vi "Control_2.vi"(0 "latd-lon-heig-VNWU":T4, 1 "CIVITA as DMARS [rad]":cluster{"phi":dbl, "theta":dbl, "psi":dbl}, 5 "Wi1-Wbi1-qi1-Euli1":T5, 7 "Civita?":bool, 9 "Mab":T3, 11 "File":dbl[][](array[numeric]), 12 "dt-sim_run-t-i":T2, 14 "Rotation":T1, 15 "sim_running":bool) -> (3 "Pitch Yaw ref [deg]":dbl[](array[numeric]), 4 "TVA_cmd(i+1,:) [deg]":dbl[](array[numeric]), 10 "AoA-Speed-Rocket":cluster{dbl[], dbl[], dbl[]})   [LabVIEW 2017]
uses:
  <vilib>/Analysis/coordinate.llb/Euler Rotation Order.ctl
  <vilib>/Analysis/_algsub.llb/Vector Norm Type.ctl
  <vilib>/Analysis/baseanly.llb/Real A x B.vi
  <vilib>/Analysis/_algsub.llb/Real Vector Norm.vi
  <vilib>/Analysis/Matrix/Numeric/Conversions/Array To Matrix - RA2.vi
  <vilib>/Analysis/Matrix/Numeric/Conversions/Matrix To Array - RM.vi
  <vilib>/Analysis/NI_AALPro.lvlib
  <vilib>/Analysis/Matrix/NI_Matrix.lvlib
  <vilib>/Analysis/NI_AALBase.lvlib
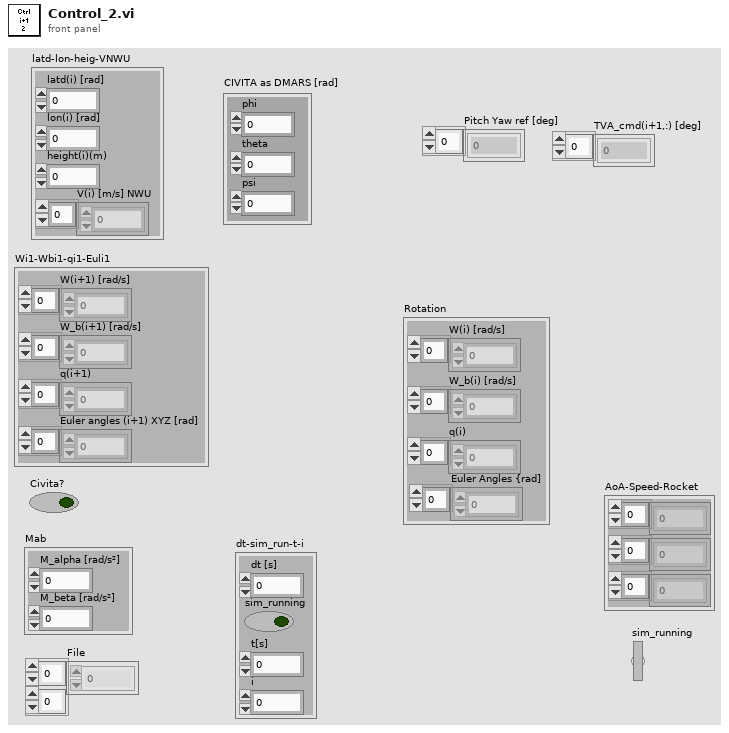
[diagram p1: front panel]
types:
  T1 = cluster{"W(i) [rad/s]":dbl[], "W_b(i) [rad/s]":dbl[], "q(i)":dbl[], "Euler Angles {rad]":dbl[]}
  T2 = cluster{"dt [s]":dbl, "sim_running":bool, "t[s]":dbl, "i":i32}
  T3 = cluster{"M_alpha [rad/s²]":dbl, "M_beta [rad/s²]":dbl}
  T4 = cluster{"latd(i) [rad]":dbl, "lon(i) [rad]":dbl, "height(i)(m)":dbl, "V(i) [m/s] NWU":dbl[]}
  T5 = cluster{"W(i+1) [rad/s]":dbl[], "W_b(i+1) [rad/s]":dbl[], "q(i+1)":dbl[], "Euler angles (i+1) XYZ [rad]":dbl[]}
  T6 = typedef "NI_AALPro.lvlib/Vector Norm Type.ctl" = u16
  T7 = typedef "NI_AALPro.lvlib/Euler Rotation Order.ctl" = u16
  T8 = typedef "NI_Matrix.lvlib/RealMatrix.ctl" = dbl[][]
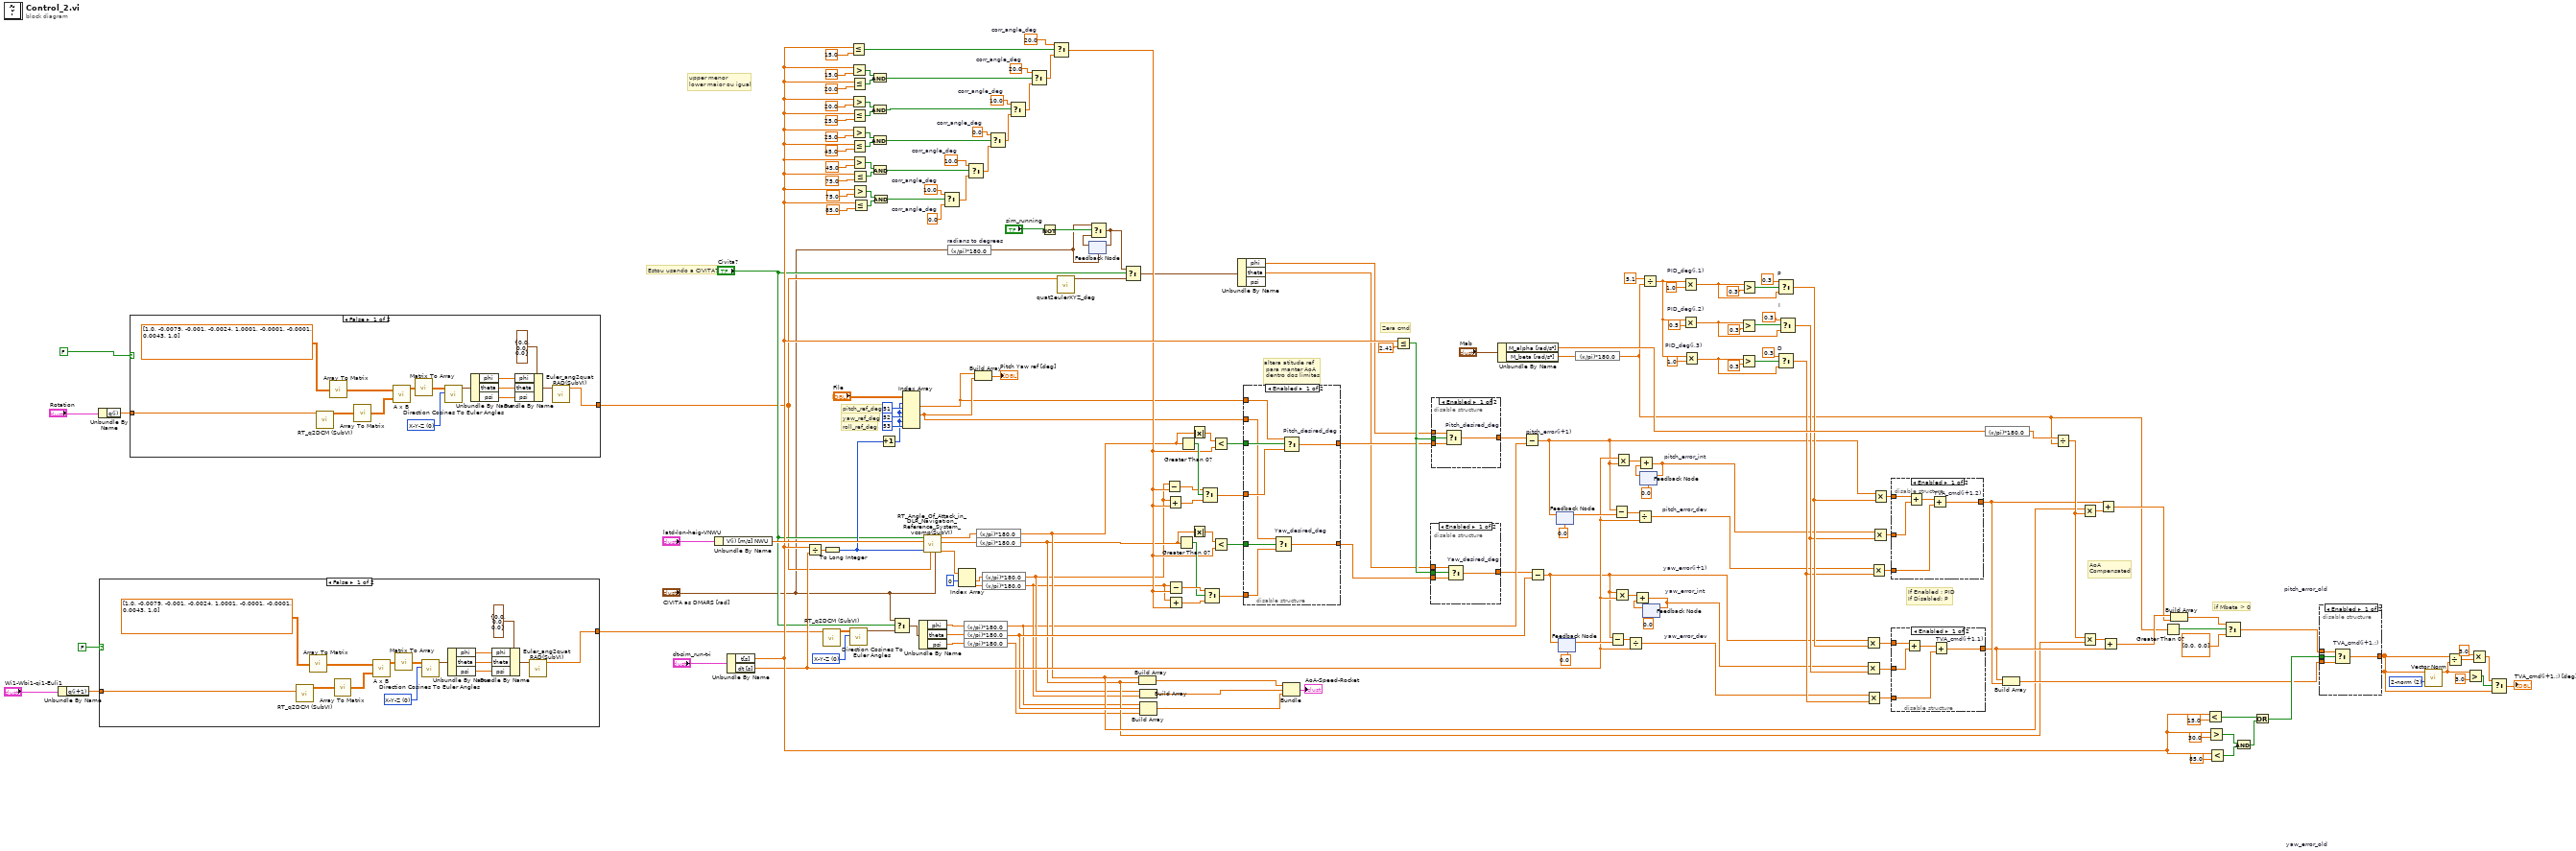
[diagram p0: block diagram]
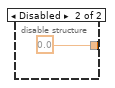
[diagram p5: hidden frame]
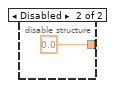
[diagram p8: hidden frame]
diagram:
  w116 = T6 2 items=["1-norm"=1, "2-norm"=2, "Inf-norm"=3, "-Inf-norm"=4, "User Defined"=5] ("norm type")
  w147 = T7 0 items=["X-Y-Z", "X-Z-Y", "Y-X-Z", "Y-Z-X", "Z-X-Y", "Z-Y-X", "X-Y-X", "X-Z-X", "Y-X-Y", "Y-Z-Y", "Z-X-Z", "Z-Y-Z"] ("rotation order")
  w156 = 0.0  # corr_angle_deg
  w159 = 10.0  # corr_angle_deg
  w162 = 10.0  # corr_angle_deg
  w187 = 0.0  # corr_angle_deg
  w189 = 10.0  # corr_angle_deg
  w191 = 20.0  # corr_angle_deg
  w192 = 20.0  # corr_angle_deg
  # "AoA\nCompensated"
  # "Estou usando a CIVITA?"
  # "If Enabled : PID\nIf Disabled: P"
  # "if Mbeta > 0"
  # "altera atitude ref\n para manter AoA\n dentro dos limites"
  # "Zera cmd"
  # "roll_ref_deg"
  # "yaw_ref_deg"
  # "pitch_ref_deg"
  # "upper menor\nlower maior ou igual"
  n1 = Unbundle By Name("Wi1-Wbi1-qi1-Euli1") -> ("q(i+1)"=w8:dbl[])
  n2 = Unbundle By Name("Rotation") -> ("q(i)"=w13:dbl[])
  n3 = case shown="False" FALSE {
    tunnel: w8 -> [w197 w210]
    tunnel: [w196 w210] -> w7
    frame False {
      w208 = T7 0 items=["X-Y-Z", "X-Z-Y", "Y-X-Z", "Y-Z-X", "Z-X-Y", "Z-Y-X", "X-Y-X", "X-Z-X", "Y-X-Y", "Y-Z-Y", "Z-X-Z", "Z-Y-Z"] ("rotation order")
      n4 = call "RT_q2DCM (SubVI).vi"("Quaternion"=w197) -> ("DCM"=w209:dbl[][])  [unwired: 10 in]
      n5 = call-poly <vilib>:"Array To Matrix.vi"("Real 2D Array"=dbl[][] [[1.0, -0.0079, -0.001], [-0.0024, 1.0001, -0.0001], [-0.0001, 0.0043, 1.0]]) -> ("Real Matrix"=w200:T8)
      n6 = call-poly <vilib>:"Array To Matrix.vi"("Real 2D Array"=w209) -> ("Real Matrix"=w199:T8)
      n7 = call-poly <vilib>:"A x B.vi"("B"=w199, "A"=w200) -> ("A x B"=w201:T8)  [unwired: 1 out]
      n8 = call-poly <vilib>:"Matrix To Array.vi"("Real Matrix"=w201) -> ("Real 2D Array"=w202:dbl[][])
      n9 = call <vilib>:"Direction Cosines To Euler Angles.vi"("rotation order"=w208, "Direction Cosines"=w202) -> ("Euler Angles"=w203:cluster{"phi":dbl, "theta":dbl, "psi":dbl})  [unwired: 8 in, 1 out]
      n10 = Unbundle By Name(w203) -> ("phi"=w206:dbl, "theta"=w207:dbl, "psi"=w195:dbl)
      n11 = Bundle By Name(cluster=cluster{"phi":dbl, "theta":dbl, "psi":dbl} {"phi"=0.0, "theta"=0.0, "psi"=0.0} ("Euler Angles 2"), "phi"=w206, "theta"=w207, "psi"=w195) -> (w204:cluster{"phi":dbl, "theta":dbl, "psi":dbl})
      n12 = call "Euler_ang2quat RAD(SubVI).vi"("Euler Angles [rad]"=w204) -> ("Quaternions"=w196:dbl[])  [unwired: 10 in]
    }
    frame True {
    }
  }
  n13 = case shown="False" FALSE {
    tunnel: w13 -> [w213 w226]
    tunnel: [w212 w226] -> w11
    frame False {
      w224 = T7 0 items=["X-Y-Z", "X-Z-Y", "Y-X-Z", "Y-Z-X", "Z-X-Y", "Z-Y-X", "X-Y-X", "X-Z-X", "Y-X-Y", "Y-Z-Y", "Z-X-Z", "Z-Y-Z"] ("rotation order")
      n14 = call "RT_q2DCM (SubVI).vi"("Quaternion"=w213) -> ("DCM"=w225:dbl[][])  [unwired: 10 in]
      n15 = call-poly <vilib>:"Array To Matrix.vi"("Real 2D Array"=dbl[][] [[1.0, -0.0079, -0.001], [-0.0024, 1.0001, -0.0001], [-0.0001, 0.0043, 1.0]]) -> ("Real Matrix"=w216:T8)
      n16 = call-poly <vilib>:"Array To Matrix.vi"("Real 2D Array"=w225) -> ("Real Matrix"=w215:T8)
      n17 = call-poly <vilib>:"A x B.vi"("B"=w215, "A"=w216) -> ("A x B"=w217:T8)  [unwired: 1 out]
      n18 = call-poly <vilib>:"Matrix To Array.vi"("Real Matrix"=w217) -> ("Real 2D Array"=w218:dbl[][])
      n19 = call <vilib>:"Direction Cosines To Euler Angles.vi"("rotation order"=w224, "Direction Cosines"=w218) -> ("Euler Angles"=w219:cluster{"phi":dbl, "theta":dbl, "psi":dbl})  [unwired: 8 in, 1 out]
      n20 = Unbundle By Name(w219) -> ("phi"=w222:dbl, "theta"=w223:dbl, "psi"=w211:dbl)
      n21 = Bundle By Name(cluster=cluster{"phi":dbl, "theta":dbl, "psi":dbl} {"phi"=0.0, "theta"=0.0, "psi"=0.0} ("Euler Angles 2"), "phi"=w222, "theta"=w223, "psi"=w211) -> (w220:cluster{"phi":dbl, "theta":dbl, "psi":dbl})
      n22 = call "Euler_ang2quat RAD(SubVI).vi"("Euler Angles [rad]"=w220) -> ("Quaternions"=w212:dbl[])  [unwired: 10 in]
    }
    frame True {
    }
  }
  n23 = Unbundle By Name("latd-lon-heig-VNWU") -> ("V(i) [m/s] NWU"=w83:dbl[])
  n24 = Unbundle By Name("dt-sim_run-t-i") -> ("t[s]"=w77:dbl, "dt [s]"=w58:dbl)
  n25 = Divide(x=w77, y=w58) -> (x/y=w154:dbl)
  n26 = call "RT_q2DCM (SubVI).vi"("Quaternion"=w7) -> ("DCM"=w148:dbl[][])  [unwired: 10 in]
  n27 = To Long Integer(number=w154) -> (32bit integer=w72:i32)
  n28 = Less Or Equal?(x=w77, y=15.0) -> (x <= y?=w193:bool)
  n29 = call <vilib>:"Direction Cosines To Euler Angles.vi"("rotation order"=w147, "Direction Cosines"=w148) -> ("Euler Angles"=w6:cluster{"phi":dbl, "theta":dbl, "psi":dbl})  [unwired: 8 in, 1 out]
  n30 = Greater?(x=w77, y=15.0) -> (0:w183:bool)
  n31 = Greater?(x=w77, y=20.0) -> (0:w179:bool)
  n32 = Greater?(x=w77, y=25.0) -> (0:w174:bool)
  n33 = Less Or Equal?(x=w77, y=20.0) -> (x <= y?=w182:bool)
  n34 = Less Or Equal?(x=w77, y=25.0) -> (x <= y?=w180:bool)
  n35 = Less Or Equal?(x=w77, y=45.0) -> (x <= y?=w173:bool)
  n36 = Greater?(x=w77, y=45.0) -> (0:w171:bool)
  n37 = Less Or Equal?(x=w77, y=75.0) -> (x <= y?=w172:bool)
  n38 = Greater?(x=w77, y=75.0) -> (0:w166:bool)
  n39 = Less Or Equal?(x=w77, y=85.0) -> (x <= y?=w165:bool)
  n40 = And(x=w183, y=w182) -> (x .and. y?=w181:bool)
  n41 = And(x=w179, y=w180) -> (x .and. y?=w164:bool)
  n42 = And(x=w174, y=w173) -> (x .and. y?=w163:bool)
  n43 = And(x=w171, y=w172) -> (x .and. y?=w161:bool)
  n44 = And(x=w166, y=w165) -> (x .and. y?=w158:bool)
  n45 = Increment(x=w72) -> (x+1=w144:i32)
  n46 = Select(t="CIVITA as DMARS [rad]", s="Civita?", f=w6) -> (s? t:f=w31:cluster{"phi":dbl, "theta":dbl, "psi":dbl})
  n47 = Index Array(array="File", index (row) #1=w144, index (col) #1=51 ("disabled index (col)"), index (row) #2=w144, index (col) #2=52 ("disabled index (col)"), index (row) #3=w144, index (col) #3=53 ("disabled index (col)")) -> (element #1=w36:dbl, element #2=w37:dbl)  [unwired: 1 out]
  n48 = Unbundle By Name(w31) -> ("phi"=w146:dbl, "theta"=w145:dbl, "psi"=w35:dbl)
  n49 = call "RT_Angle_Of_Attack_in_DLR_Navigation_Reference_System_vcomp(SubVI).vi"("Euler Angles [rad]"="CIVITA as DMARS [rad]", "q"=w11, "i"=w72, "V (m/s)"=w83, "Civita?"="Civita?") -> ("Speed_direction [rad]"=w149:dbl[], "AoA_yaw (rad)"=w42:dbl, "AoA_pitch (rad)"=w43:dbl)  [unwired: 4 in]
  n50 = Select(t=w159, s=w158, f=w156) -> (s? t:f=w157:dbl)
  n51 = expression code="(x/pi)*180.0" "radians to degrees"("CIVITA as DMARS [rad]") -> (w17:cluster{"phi":dbl, "theta":dbl, "psi":dbl})
  n52 = Index Array(array=w149, index #1=0 ("index")) -> (element #1=w45:dbl, element #2=w44:dbl)  [unwired: 1 in]
  n53 = expression code="(x/pi)*180.0" ("radians to degrees")(w146) -> (w26:dbl)
  n54 = expression code="(x/pi)*180.0" ("radians to degrees")(w145) -> (w46:dbl)
  n55 = expression code="(x/pi)*180.0" ("radians to degrees")(w35) -> (w34:dbl)
  n56 = Select(t=w162, s=w161, f=w157) -> (s? t:f=w160:dbl)
  n57 = Build Array(w36, w37) -> (→"Pitch Yaw ref [deg]":dbl[])
  n58 = expression code="(x/pi)*180.0" ("radians to degrees")(w43) -> (w41:dbl)
  n59 = expression code="(x/pi)*180.0" ("radians to degrees")(w42) -> (w40:dbl)
  n60 = expression code="(x/pi)*180.0" ("radians to degrees")(w45) -> (w39:dbl)
  n61 = expression code="(x/pi)*180.0" ("radians to degrees")(w44) -> (w38:dbl)
  n62 = Select(t=w187, s=w163, f=w160) -> (s? t:f=w186:dbl)
  n63 = Select(t=w189, s=w164, f=w186) -> (s? t:f=w188:dbl)
  n64 = Select(t=w191, s=w181, f=w188) -> (s? t:f=w190:dbl)
  n65 = Not(x="sim_running") -> (.not. x?=w21:bool)
  n66 = Select(t=w192, s=w193, f=w190) -> (s? t:f=w71:dbl)
  n67 = call "quat2eulerXYZ_deg.vi"("Quaternions"=w11) -> ("Euler Angles [deg]"=w30:cluster{"phi":dbl, "theta":dbl, "psi":dbl})  [unwired: 10 in]
  n68 = feedback #1(w17) -> (w27:cluster{"phi":dbl, "theta":dbl, "psi":dbl})
  n69 = Select(t=w17, s=w21, f=w27) -> (s? t:f=w32:cluster{"phi":dbl, "theta":dbl, "psi":dbl})
  n70 = feedback-in #1(w32) -> ()
  n71 = Select(t=w32, s="Civita?", f=w30) -> (s? t:f=w29:cluster{"phi":dbl, "theta":dbl, "psi":dbl})
  n72 = Build Array(w41, w40) -> (w16:dbl[])
  n73 = Build Array(w39, w38) -> (w15:dbl[])
  n74 = Build Array(w26, w46, w34) -> (w14:dbl[])
  n75 = Subtract(x=w39, y=w71) -> (x-y=w104:dbl)
  n76 = Add(x=w39, y=w71) -> (x+y=w103:dbl)
  n77 = Subtract(x=w38, y=w71) -> (x-y=w101:dbl)
  n78 = Add(x=w38, y=w71) -> (x+y=w102:dbl)
  n79 = Greater Than 0?(x=w40) -> (x > 0?=w100:bool)
  n80 = Greater Than 0?(x=w41) -> (x > 0?=w105:bool)
  n81 = Absolute Value(x=w41) -> (abs(x)=w108:dbl)
  n82 = Absolute Value(x=w40) -> (abs(x)=w97:dbl)
  n83 = Select(t=w104, s=w105, f=w103) -> (s? t:f=w106:dbl)
  n84 = Select(t=w101, s=w100, f=w102) -> (s? t:f=w99:dbl)
  n85 = Less?(x=w108, y=w71) -> (x < y?=w107:bool)
  n86 = Less?(x=w97, y=w71) -> (x < y?=w98:bool)
  n87 = Unbundle By Name(w29) -> ("phi"=w19:dbl, "theta"=w18:dbl)  [unwired: 1 out]
  n88 = disable-structure shown="Enabled" {
    disable-tunnel: w37 -> [w228 w235]
    disable-tunnel: w36 -> [w230 w236]
    disable-tunnel: w107 -> [w234 _]
    disable-tunnel: w106 -> [w229 _]
    disable-tunnel: w99 -> [w227 _]
    disable-tunnel: w98 -> [w231 _]
    disable-tunnel: [w233 w236] -> w94
    disable-tunnel: [w232 w235] -> w93
    frame Enabled {
      n89 = Select "Yaw_desired_deg"(t=w228, s=w231, f=w227) -> (s? t:f=w232:dbl)
      n90 = Select "Pitch_desired_deg"(t=w230, s=w234, f=w229) -> (s? t:f=w233:dbl)
    }
    frame Disabled {
    }
  }
  n91 = Bundle(w16, w15, w14) -> (→"AoA-Speed-Rocket":cluster{dbl[], dbl[], dbl[]})  [unwired: 1 in]
  n92 = Less Or Equal?(x=w77, y=2.41) -> (x <= y?=w95:bool)
  n93 = disable-structure shown="Enabled" {
    disable-tunnel: [w240 0.0 ("t")] -> w24
    disable-tunnel: w95 -> [w237 _]
    disable-tunnel: w93 -> [w239 _]
    disable-tunnel: w18 -> [w238 _]
    frame Enabled {
      n94 = Select "Yaw_desired_deg"(t=w238, s=w237, f=w239) -> (s? t:f=w240:dbl)
    }
    frame Disabled {
    }
  }
  n95 = disable-structure shown="Enabled" {
    disable-tunnel: [w245 0.0 ("t")] -> w25
    disable-tunnel: w95 -> [w244 _]
    disable-tunnel: w94 -> [w243 _]
    disable-tunnel: w19 -> [w242 _]
    frame Enabled {
      n96 = Select "Pitch_desired_deg"(t=w242, s=w244, f=w243) -> (s? t:f=w245:dbl)
    }
    frame Disabled {
    }
  }
  n97 = Unbundle By Name("Mab") -> ("M_alpha [rad/s²]"=w81:dbl, "M_beta [rad/s²]"=w79:dbl)
  n98 = Subtract "pitch_error(i+1)"(x=w25, y=w26) -> (x-y=w23:dbl)
  n99 = Subtract "yaw_error(i+1)"(x=w24, y=w46) -> (x-y=w22:dbl)
  n100 = feedback #2 "pitch_error_old"(0.0) -> (w92:dbl)
  n101 = feedback-in #2(w23) -> ()
  n102 = feedback #3 "yaw_error_old"(0.0) -> (w90:dbl)
  n103 = feedback-in #3(w22) -> ()
  n104 = expression code="(x/pi)*180.0" ("radians to degrees")(w79) -> (w3:dbl)
  n105 = Subtract ("yaw_error_dev")(x=w22, y=w90) -> (x-y=w89:dbl)
  n106 = Subtract ("pitch_error_dev")(x=w23, y=w92) -> (x-y=w91:dbl)
  n107 = Multiply(x=w22, y=w58) -> (x*y=w57:dbl)
  n108 = Multiply(x=w58, y=w23) -> (x*y=w54:dbl)
  n109 = Divide "yaw_error_dev"(x=w89, y=w58) -> (x/y=w60:dbl)
  n110 = Divide "pitch_error_dev"(x=w91, y=w58) -> (x/y=w62:dbl)
  n111 = feedback #4(0.0) -> (w55:dbl)
  n112 = Add "pitch_error_int"(x=w54, y=w55) -> (x+y=w59:dbl)
  n113 = feedback-in #4(w59) -> ()
  n114 = Divide(x=5.1, y=w3) -> (x/y=w136:dbl)
  n115 = feedback #5(0.0) -> (w56:dbl)
  n116 = Add "yaw_error_int"(x=w57, y=w56) -> (x+y=w61:dbl)
  n117 = feedback-in #5(w61) -> ()
  n118 = Multiply "PID_deg(i,1)"(x=w136, y=1.0) -> (x*y=w132:dbl)
  n119 = Multiply "PID_deg(i,2)"(x=w136, y=0.5) -> (x*y=w127:dbl)
  n120 = Multiply "PID_deg(i,3)"(x=w136, y=1.0) -> (x*y=w126:dbl)
  n121 = Greater?(x=w127, y=0.3) -> (0:w128:bool)
  n122 = Greater?(x=w126, y=0.3) -> (0:w129:bool)
  n123 = Greater?(x=w132, y=0.3) -> (0:w134:bool)
  n124 = Select "P"(t=0.3, s=w134, f=w132) -> (s? t:f=w70:dbl)
  n125 = Select "D"(t=0.3, s=w129, f=w126) -> (s? t:f=w66:dbl)
  n126 = Select "I"(t=0.3, s=w128, f=w127) -> (s? t:f=w67:dbl)
  n127 = Multiply(x=w22, y=w70) -> (x*y=w68:dbl)
  n128 = Multiply(x=w61, y=w67) -> (x*y=w65:dbl)
  n129 = Multiply(x=w60, y=w66) -> (x*y=w64:dbl)
  n130 = Multiply(x=w62, y=w66) -> (x*y=w69:dbl)
  n131 = Multiply(x=w59, y=w67) -> (x*y=w124:dbl)
  n132 = Multiply(x=w23, y=w70) -> (x*y=w125:dbl)
  n133 = disable-structure shown="Enabled" {
    disable-tunnel: w125 -> [w251 w252]
    disable-tunnel: w124 -> [w247 _]
    disable-tunnel: [w249 w252] -> w87
    disable-tunnel: w69 -> [w248 _]
    frame Enabled {
      n134 = Add(x=w251, y=w247) -> (x+y=w250:dbl)
      n135 = Add "TVA_cmd(i+1,2)"(x=w250, y=w248) -> (x+y=w249:dbl)
    }
    frame Disabled {
    }
  }
  n136 = disable-structure shown="Enabled" {
    disable-tunnel: w68 -> [w257 w258]
    disable-tunnel: w65 -> [w253 _]
    disable-tunnel: [w255 w258] -> w63
    disable-tunnel: w64 -> [w254 _]
    frame Enabled {
      n137 = Add(x=w257, y=w253) -> (x+y=w256:dbl)
      n138 = Add "TVA_cmd(i+1,1)"(x=w256, y=w254) -> (x+y=w255:dbl)
    }
    frame Disabled {
    }
  }
  n139 = expression code="(x/pi)*180.0" ("radians to degrees")(w81) -> (w80:dbl)
  n140 = Build Array(w63, w87) -> (w48:dbl[])
  n141 = Divide(x=w80, y=w3) -> (x/y=w118:dbl)
  n142 = Multiply(x=w41, y=w118) -> (x*y=w2:dbl)
  n143 = Multiply(x=w118, y=w40) -> (x*y=w1:dbl)
  n144 = Add(x=w87, y=w2) -> (x+y=w85:dbl)
  n145 = Add(x=w1, y=w63) -> (x+y=w86:dbl)
  n146 = Greater Than 0?(x=w3) -> (x > 0?=w120:bool)
  n147 = Build Array(w86, w85) -> (w117:dbl[])
  n148 = Less?(x=w77, y=15.0) -> (x < y?=w51:bool)
  n149 = Greater?(x=w77, y=30.0) -> (0:w53:bool)
  n150 = Less?(x=w77, y=85.0) -> (x < y?=w52:bool)
  n151 = Select(t=w117, s=w120, f=dbl[] [0.0, 0.0] ("appended array")) -> (s? t:f=w75:dbl[])
  n152 = And(x=w53, y=w52) -> (x .and. y?=w50:bool)
  n153 = Or(x=w51, y=w50) -> (x .or. y?=w49:bool)
  n154 = disable-structure shown="Enabled" {
    disable-tunnel: w49 -> [w262 _]
    disable-tunnel: w75 -> [w261 _]
    disable-tunnel: w48 -> [w260 w263]
    disable-tunnel: [w259 w263] -> w88
    frame Enabled {
      n155 = Select "TVA_cmd(i+1,:)"(t=w261, s=w262, f=w260) -> (s? t:f=w259:dbl[])
    }
    frame Disabled {
    }
  }
  n156 = call-poly <vilib>:"Vector Norm.vi"("norm type"=w116, "Input Vector"=w88) -> ("norm"=w113:dbl)  [unwired: 8 in, 1 out]
  n157 = Divide(x=w88, y=w113) -> (x/y=w111:dbl[])
  n158 = Greater?(x=w113, y=3.0) -> (0:w114:bool)
  n159 = Multiply(x=3.0, y=w111) -> (x*y=w110:dbl[])
  n160 = Select(t=w110, s=w114, f=w88) -> (s? t:f=→"TVA_cmd(i+1,:) [deg]":dbl[])
